vi "Holding Register Set DataType.vi"(8 "error in (no error)":errorcluster, 10 "DataType":T1, 11 "Item Ref in":T2 format="%.0x") -> (0 "error out":errorcluster, 3 "Item Ref out":T2 format="%.0x")   [LabVIEW 2021]
uses:
  <vilib>/NI VeriStand/Custom Device API/Custom Device API.lvlib
  Shared/Constants.vi
  Shared/Modbus Master Shared.lvlib
  <vilib>/NI VeriStand/Custom Device API/Set Item Property (U16).vi
  <vilib>/NI VeriStand/Custom Device API/Custom Device Item Ref.ctl
  Shared/Controls/Data Model/DataType.ctl
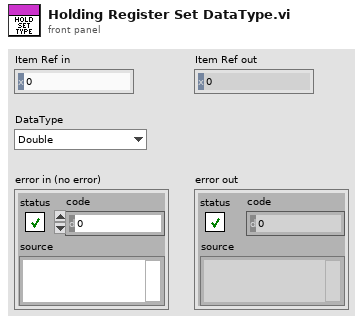
[diagram p1: front panel]
types:
  T1 = typedef "Modbus Master Shared.lvlib/DataType.ctl" = enum16{"Double", "Single", "I64", "I32", "I16", "I8", "U64", "U32", "U16", "U8", "Boolean"}
  T2 = typedef "Custom Device API.lvlib/Custom Device Item Ref.ctl" = u64
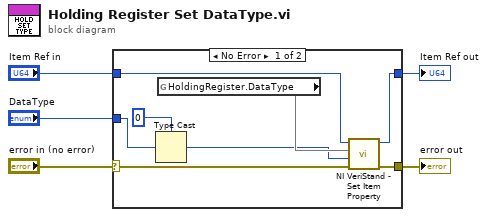
[diagram p0: block diagram]
diagram:
  n1 = case shown="No Error" "error in (no error)" {
    selector: "error in (no error)" -> [w12 w14]
    tunnel: "Item Ref in" -> [w11 w15]
    tunnel: [w10 w14] -> w3
    tunnel: [w9 w15] -> w2
    tunnel: "DataType" -> [w6 _]
    frame No Error {
      n2 = Type Cast(type=u16 0, x=w6) -> (*(type *) &x=w7:u16)
      n3 = global read "Constants.vi" "HoldingRegister.DataType"() -> (w13)
      n4 = call-poly <vilib>:"NI VeriStand - Set Item Property.vi"("error in (no error)"=w12, "Value"=w7, "Property Name"=w13, "Item Ref in"=w11) -> ("error out"=w10:errorcluster, "Item Ref out"=w9:T2)  [unwired: 5 in, 1 out]
    }
    frame Error {
    }
  }
  "error out" <- w3
  "Item Ref out" <- w2
